vi "Generate MeasurementLink Server Internal.vi"(8 "error in (no error)":errorcluster) -> (0 "error out":errorcluster)   [LabVIEW 2020, in "MeasurementLink Proto Builds.lvlib"]
uses:
  MeasurementLink Proto Builds.lvlib
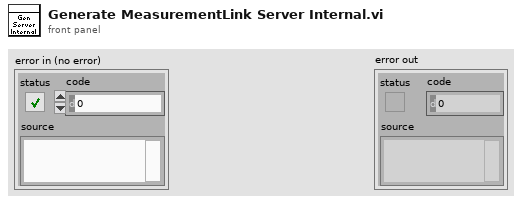
[diagram p1: front panel]
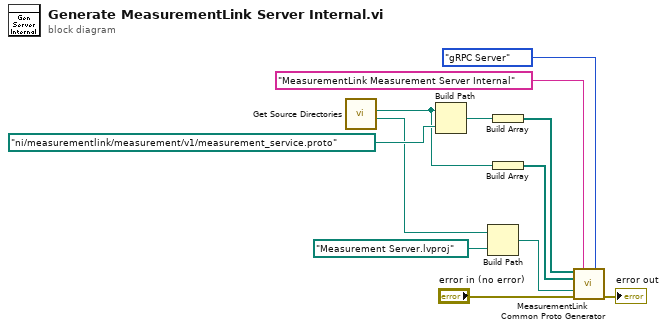
[diagram p0: block diagram]
diagram:
  n1 = call "Get Source Directories.vi"() -> ("Runtime Dir"=w1:path, "Protos Dir"=w2:path)  [unwired: 9 in, 1 out]
  n2 = Build Path(base path=w2, name or relative path=path "ni/measurementlink/measurement/v1/measurement_service.proto" ("Proto File Path")) -> (appended path=w11:path)
  n3 = Build Path(base path=w1, name or relative path=path "Measurement Server.lvproj" ("Target Project")) -> (appended path=w3:path)
  n4 = Build Array(w11) -> (w5:path[])
  n5 = Build Array(w2) -> (w6:path[])
  n6 = call "MeasurementLink Common Proto Generator.vi"("Proto File Path"=w5, "Generated Library Full Name"="MeasurementLink Measurement Server Internal" ("Generated Library Name"), "Generate"=enum16{"gRPC Server", "gRPC Client", "Both"}."gRPC Server", "Import Paths"=w6, "Target Project"=w3, "error in (no error)"="error in (no error)") -> ("error out"=→"error out":errorcluster)  [unwired: 9 in]
